vi "0037-0003_Si7021.vi"() -> ()   [LabVIEW 2014]
panel:
  out "temp 2":dbl format="%#.2g"
  out "temp":dbl format="%#.2g"
  out "x = y?":bool
  out "error out":errorcluster caption="エラー出力"
  in  "停止ボタン":bool
  # "℃"
  # "％RH"
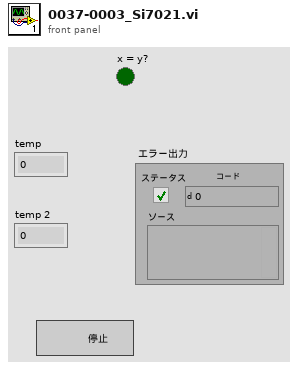
[diagram p1: front panel]
types:
  T1 = cluster{"bitRate":u32, "address":u8, "autoReadRespond":bool, "writeTimeout":u16, "readTimeout":u16, "sclLowTimeout":bool, "transferRetries":u16}
  T2 = typedef "CP2112_device.ctl" = i32
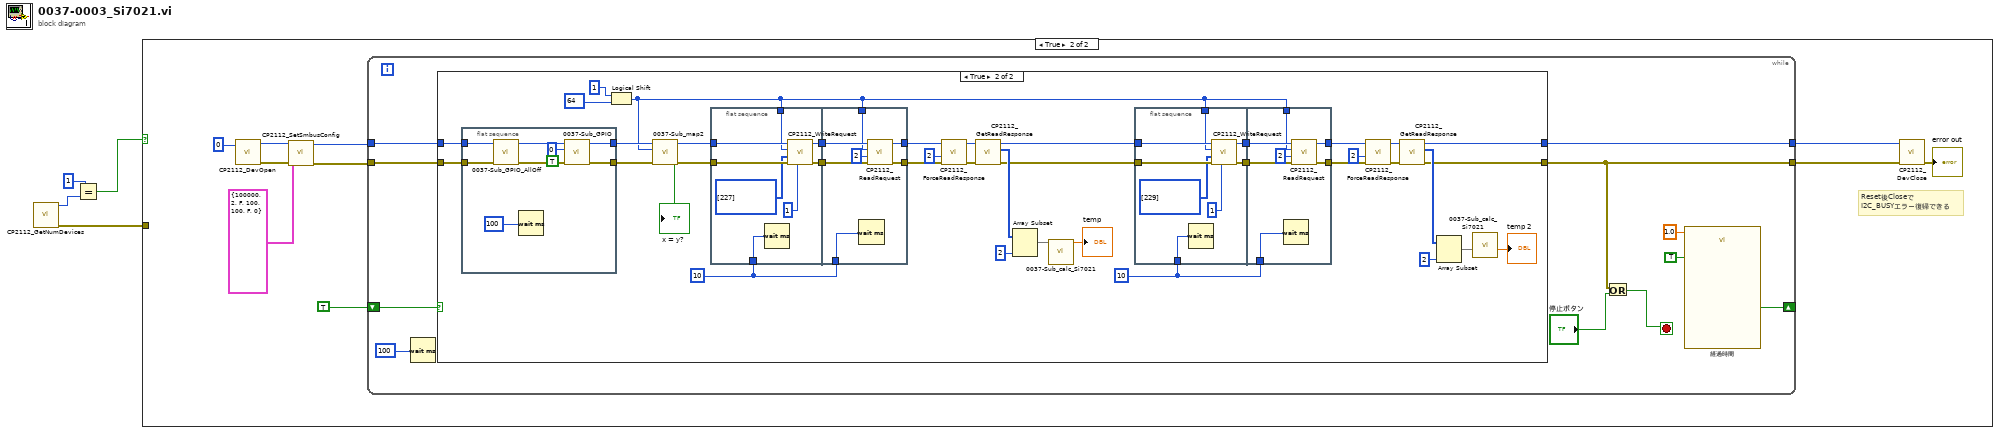
[diagram p0: block diagram]
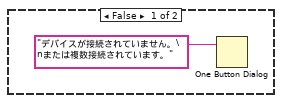
[diagram p2: hidden frame]
diagram:
  n1 = call "CP2112_GetNumDevices.vi"() -> ("error out"=w1:errorcluster, "numDevices"=w3:i32)  [unwired: 9 in, 1 out]
  n2 = Equal?(x=1, y=w3) -> (x = y?=w2:bool)
  n3 = case shown="TRUE" w2 {
    tunnel: w1 -> [_ _]
    frame False {
      n4 = One Button Dialog(message="デバイスが接続されていません。\nまたは複数接続されています。" ("メッセージ")) -> ()  [unwired: 1 in, 1 out]
    }
    frame True {
      # "Reset後Closeで\nI2C_BUSYエラー復帰できる"
      n5 = call "CP2112_DevOpen.vi"("deviceNum"=0) -> ("error out"=w10:errorcluster, "device"=w11:T2)  [unwired: 8 in, 1 out]
      n6 = call "CP2112_SetSmbusConfig.vi"("error in (no error)"=w10, "smbusInfo"=T1 {"bitRate"=100000, "address"=2, "autoReadRespond"=FALSE, "writeTimeout"=100, "readTimeout"=100, "sclLowTimeout"=FALSE, "transferRetries"=0}, "device"=w11) -> ("error out"=w12:errorcluster, "deviceOut"=w13:T2)  [unwired: 6 in, 1 out]
      n7 = while {
        tunnel: w12 -> [w26]
        tunnel: w13 -> [w25]
        tunnel: [w22] -> w8
        tunnel: [w21] -> w7
        shift-right: [w18] -> _
        shift-left: TRUE ("Auto Reset") -> [w19]
        stop <- w23 stop-if-true
        n8 = Wait (ms)(milliseconds to wait=u32 100 ("ミリ秒待機時間")) -> ()  [unwired: 1 out]
        n9 = case shown="TRUE" w19 {
          tunnel: w26 -> [w27 w55]
          tunnel: w25 -> [w28 w56]
          tunnel: [w27 w32] -> w22
          tunnel: [w28 w33] -> w21
          frame False {
          }
          frame True {
            w36 = u32 10 ("ミリ秒待機時間")
            w57 = u32 10 ("ミリ秒待機時間")
            n10 = flat-sequence {
              tunnel: w56 -> [w90]
              tunnel: w55 -> [w87]
              tunnel: [w88] -> w50
              tunnel: [w85] -> w49
              frame #0 {
                n11 = call "0037-Sub_GPIO_AllOff.vi"("エラー出力 2"=w87, "device"=w90) -> ("エラー出力"=w86:errorcluster, "deviceOut"=w89:T2)  [unwired: 8 in]
                n12 = Wait (ms)(milliseconds to wait=u32 100 ("ミリ秒待機時間")) -> ()  [unwired: 1 out]
                n13 = call "0037-Sub_GPIO.vi"("エラー出力 2"=w86, "ブール"=TRUE, "GPIO"=u8 0, "device"=w89) -> ("エラー出力"=w85:errorcluster, "deviceOut"=w88:T2)  [unwired: 6 in]
              }
            }
            n14 = Logical Shift(y=1, x=64) -> (x << y=w31:i32)
            n15 = call "0037-Sub_map2.vi"("error out"=w49, "アドレス"=w31, "device"=w50) -> ("error out 2"=w52:errorcluster, "x = y?"=→"x = y?":bool, "device 2"=w51:T2)  [unwired: 5 in]
            n16 = flat-sequence {
              tunnel: w52 -> [w98]
              tunnel: w51 -> [w97]
              tunnel: w31 -> [w92]
              tunnel: [w96] -> w61
              tunnel: [w95] -> w60
              tunnel: w57 -> [w91]
              tunnel: w61 -> [w103]
              tunnel: w60 -> [w102]
              tunnel: [w104] -> w59
              tunnel: [w101] -> w58
              tunnel: w31 -> [w100]
              tunnel: w57 -> [w99]
              frame #0 {
                n17 = Wait (ms)(milliseconds to wait=w91) -> ()  [unwired: 1 out]
                n18 = call "CP2112_WriteRequest.vi"("numBytesToWrite"=i16 1 ("numByteToRead"), "error in (no error)"=w98, "buffer"=u8[] [227], "slaveAddress"=w92, "device"=w97) -> ("error out"=w96:errorcluster, "deviceOut"=w95:T2)  [unwired: 4 in, 1 out]
              }
              frame #1 {
                n19 = Wait (ms)(milliseconds to wait=w99) -> ()  [unwired: 1 out]
                n20 = call "CP2112_ReadRequest.vi"("error in (no error)"=w103, "numByteToRead"=i16 2, "slaveAddress"=w100, "device"=w102) -> ("error out"=w104:errorcluster, "deviceOut"=w101:T2)  [unwired: 5 in, 1 out]
              }
            }
            n21 = call "CP2112_ForceReadResponse.vi"("error in (no error)"=w59, "numByteToRead"=i16 2, "device"=w58) -> ("error out"=w66:errorcluster, "deviceOut"=w65:T2)  [unwired: 6 in, 1 out]
            n22 = call "CP2112_GetReadResponse.vi"("error in (no error)"=w66, "device"=w65) -> ("error out"=w34:errorcluster, "buffer"=w63:u8[], "deviceOut"=w35:T2)  [unwired: 4 in, 3 out]
            n23 = Array Subset(array=w63, length=2 ("長さ")) -> (w47:u8[])  [unwired: 1 in]
            n24 = call "0037-Sub_calc_Si7021.vi"("temp"=w47) -> ("temp"=→"temp":dbl)  [unwired: 8 in, 1 out]
            n25 = flat-sequence {
              tunnel: w34 -> [w74]
              tunnel: w35 -> [w73]
              tunnel: w31 -> [w68]
              tunnel: [w72] -> w45
              tunnel: [w71] -> w44
              tunnel: w36 -> [w67]
              tunnel: w45 -> [w79]
              tunnel: w44 -> [w78]
              tunnel: [w80] -> w38
              tunnel: [w77] -> w37
              tunnel: w31 -> [w76]
              tunnel: w36 -> [w75]
              frame #0 {
                n26 = Wait (ms)(milliseconds to wait=w67) -> ()  [unwired: 1 out]
                n27 = call "CP2112_WriteRequest.vi"("numBytesToWrite"=i16 1 ("numByteToRead"), "error in (no error)"=w74, "buffer"=u8[] [229], "slaveAddress"=w68, "device"=w73) -> ("error out"=w72:errorcluster, "deviceOut"=w71:T2)  [unwired: 4 in, 1 out]
              }
              frame #1 {
                n28 = Wait (ms)(milliseconds to wait=w75) -> ()  [unwired: 1 out]
                n29 = call "CP2112_ReadRequest.vi"("error in (no error)"=w79, "numByteToRead"=i16 2, "slaveAddress"=w76, "device"=w78) -> ("error out"=w80:errorcluster, "deviceOut"=w77:T2)  [unwired: 5 in, 1 out]
              }
            }
            n30 = call "CP2112_ForceReadResponse.vi"("error in (no error)"=w38, "numByteToRead"=i16 2, "device"=w37) -> ("error out"=w43:errorcluster, "deviceOut"=w42:T2)  [unwired: 6 in, 1 out]
            n31 = call "CP2112_GetReadResponse.vi"("error in (no error)"=w43, "device"=w42) -> ("error out"=w32:errorcluster, "buffer"=w40:u8[], "deviceOut"=w33:T2)  [unwired: 4 in, 3 out]
            n32 = Array Subset(array=w40, length=2 ("長さ")) -> (w30:u8[])  [unwired: 1 in]
            n33 = call "0037-Sub_calc_Si7021.vi"("humi"=w30) -> ("humi"=→"temp 2":dbl)  [unwired: 8 in, 1 out]
          }
        }
        n34 = Or(x=w22, y="停止ボタン") -> (x .or. y?=w23:bool)
        n35 = call "経過時間"("Time Target (s)"=1.0, "Auto Reset"=TRUE) -> ("Time has Elapsed"=w18:bool)  [unwired: 10 in, 7 out]
      }
      n36 = call "CP2112_DevClose.vi"("error in (no error)"=w8, "device"=w7) -> ("error out"=→"error out":errorcluster)  [unwired: 9 in]
    }
  }
